vi "Test Calendar.vi"() -> ()   [LabVIEW 2015, in "Calendar.lvclass"]
uses:
  Calendar.lvclass
  DaysOfWeek.ctl
  Read ColorCalendarBackground.vi
  Read ColorCalendarSelectionBackground.vi
  Read ColorCalendarSelectionText.vi
  Read ColorCalendarText.vi
  Read ColorDaysOfWeekBackground.vi
  Read ColorDaysOfWeekText.vi
  Read ColorSelectorBackground.vi
  Read ColorSelectorText.vi
  Read FirstDayOfWeek.vi
  Read VisibleMonthYearSelect.vi
  Read VisibleTodaySelector.vi
  Read VisibleHorizontalLines.vi
  Read VisibleVerticalLines.vi
  Write ColorSelectorBackground.vi
  Write ColorDaysOfWeekText.vi
  Write ColorDaysOfWeekBackground.vi
  Write ColorSelectorText.vi
  Write ColorCalendarText.vi
  Write ColorCalendarBackground.vi
  Write ColorCalendarSelectionBackground.vi
  Write ColorCalendarSelectionText.vi
  Write VisibleTodaySelector.vi
  Write VisibleMonthYearSelect.vi
  Write FirstDayOfWeek.vi
  Write VisibleHorizontalLines.vi
  Write VisibleVerticalLines.vi
panel:
  in  "Veritcal Lines Visible":bool
  in  "Horizontal Lines Visible":bool
  in  "First Day Of Week":T1
  in  "Month-Year Selector Visible":bool
  in  "Today Selector Visible":bool
  in  "Calendar Selection Text":u32(colorbox)
  in  "Calendar Selection Background":u32(colorbox)
  in  "Calendar Background":u32(colorbox)
  in  "Calendar Text":u32(colorbox)
  in  "Selector Text":u32(colorbox)
  in  "Days of Week Background":u32(colorbox)
  in  "Days of Week Text":u32(colorbox)
  in  "Selector Background":u32(colorbox)
  out "Date Output":timestamp format="%<%A, \n%B %d, %Y>T"
  in  "Calendar":T2={"Calendar"=0, "Month"=0, "Year"=1905, "Today Button"=FALSE, "Previous Month"=FALSE, "Next Month"=FALSE, "Cal Overlay"=FALSE, "Year Selection Underlay"=FALSE} {"Year" min=1600 max=3000; "Month" items=["January", "February", "March", "April", "May", "June", "July", "August", "September", "October", "November", "December"]}
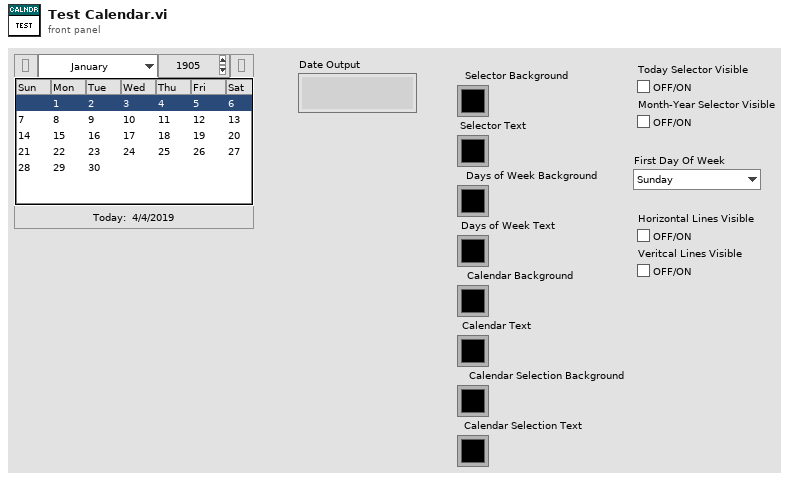
[diagram p1: front panel]
types:
  T1 = typedef "Calendar.lvclass/DaysOfWeek.ctl" = enum16{"Sunday", "Monday", "Tuesday", "Wednesday", "Thursday", "Friday", "Saturday"}
  T2 = cluster{"Calendar":i32, "Month":u16, "Year":i32, "Today Button":bool, "Previous Month":bool, "Next Month":bool, "Cal Overlay":bool, "Year Selection Underlay":bool}
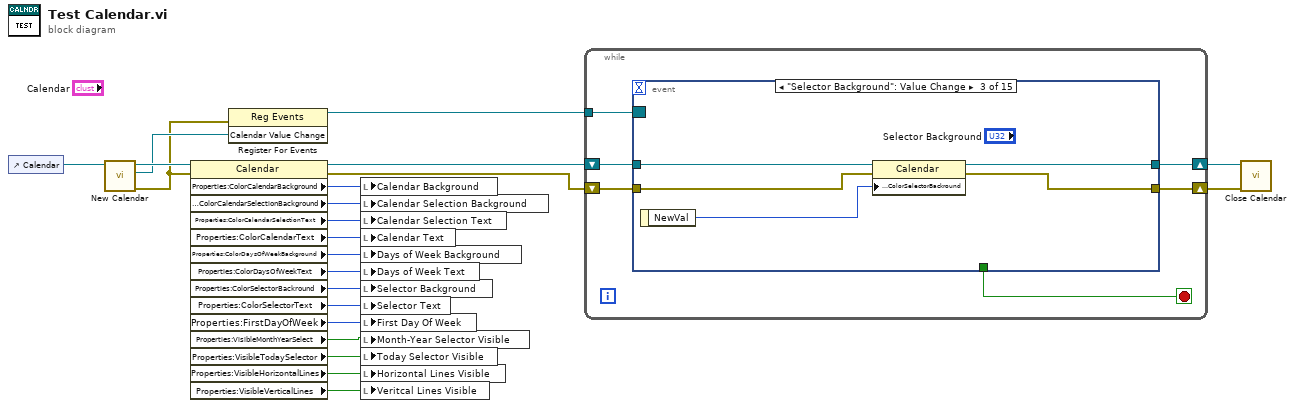
[diagram p0: block diagram]
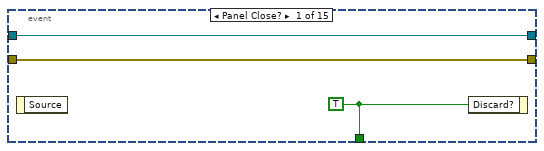
[diagram p2: hidden frame]
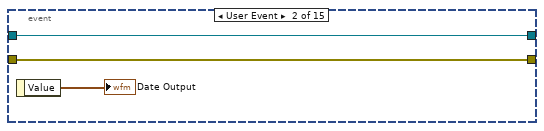
[diagram p3: hidden frame]
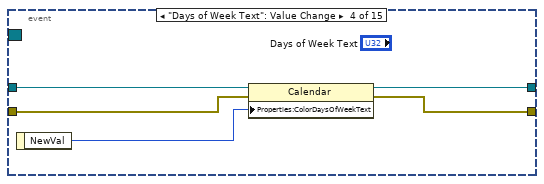
[diagram p4: hidden frame]
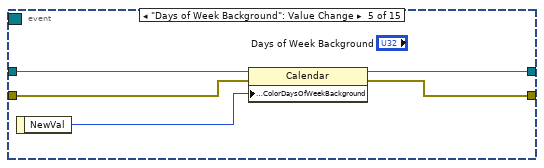
[diagram p5: hidden frame]
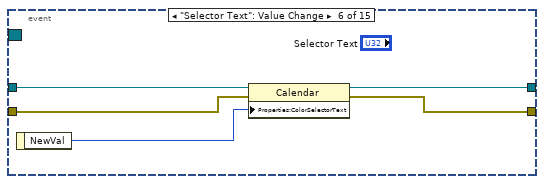
[diagram p6: hidden frame]
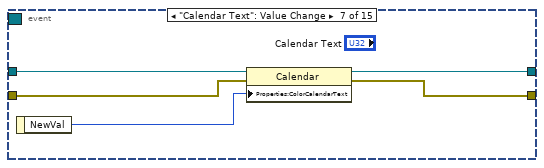
[diagram p7: hidden frame]
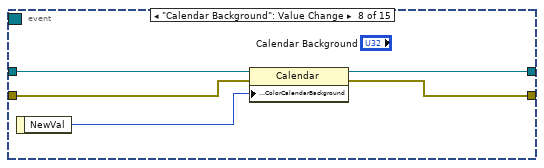
[diagram p8: hidden frame]
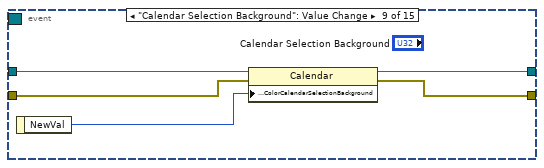
[diagram p9: hidden frame]
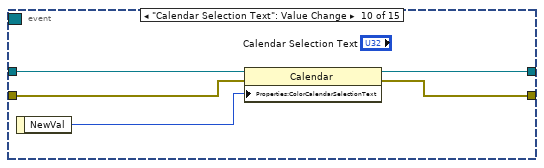
[diagram p10: hidden frame]
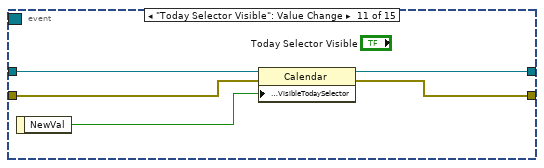
[diagram p11: hidden frame]
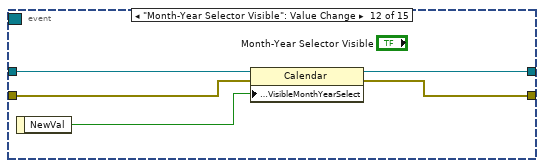
[diagram p12: hidden frame]
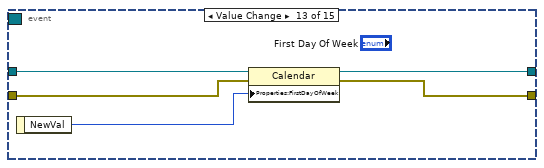
[diagram p13: hidden frame]
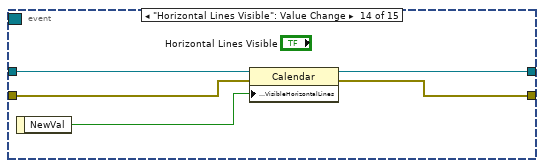
[diagram p14: hidden frame]
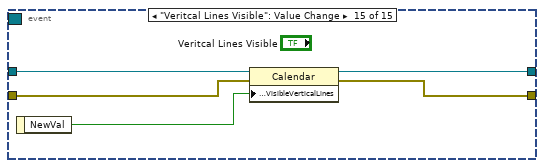
[diagram p15: hidden frame]
diagram:
  n1 = control-ref of="Calendar"() -> (w22:refnum<vi>)
  n2 = call "New Calendar.vi"("Reference"=w22) -> ("error out"=w2:errorcluster, "Calendar Value Change"=w3:refnum<user-event>, "Calendar out"=w18:refnum<class "Calendar.lvclass">)  [unwired: 8 in]
  n3 = property class="Calendar"(reference=w18, error in=w2) -> (reference out=w17:refnum<class "Calendar.lvclass">, error out=w19:errorcluster, "Properties:ColorCalendarBackground"=w16:u32, "Properties:ColorCalendarSelectionBackground"=w15:u32, "Properties:ColorCalendarSelectionText"=w14:u32, "Properties:ColorCalendarText"=w13:u32, "Properties:ColorDaysOfWeekBackground"=w12:u32, "Properties:ColorDaysOfWeekText"=w11:u32, "Properties:ColorSelectorBackround"=w10:u32, "Properties:ColorSelectorText"=w9:u32, "Properties:FirstDayOfWeek"=w8:T1, "Properties:VisibleMonthYearSelect"=w7:bool, "Properties:VisibleTodaySelector"=w6:bool, "Properties:VisibleHorizontalLines"=w5:bool, "Properties:VisibleVerticalLines"=w4:bool)
  n4 = register-events(error in=w2, w3) -> (reference out=w1:refnum<event-registration>)  [unwired: 1 in, 1 out]
  n5 = local write "Calendar Background"(w16) -> ()
  n6 = local write "Calendar Selection Background"(w15) -> ()
  n7 = local write "Calendar Selection Text"(w14) -> ()
  n8 = local write "Calendar Text"(w13) -> ()
  n9 = local write "Days of Week Background"(w12) -> ()
  n10 = local write "Days of Week Text"(w11) -> ()
  n11 = local write "Selector Background"(w10) -> ()
  n12 = local write "Selector Text"(w9) -> ()
  n13 = local write "First Day Of Week"(w8) -> ()
  n14 = local write "Month-Year Selector Visible"(w7) -> ()
  n15 = local write "Today Selector Visible"(w6) -> ()
  n16 = local write "Horizontal Lines Visible"(w5) -> ()
  n17 = local write "Veritcal Lines Visible"(w4) -> ()
  n18 = while {
    shift-right: [w27] -> w21
    shift-left: w17 -> [w26]
    shift-right: [w24] -> w20
    shift-left: w19 -> [w25]
    tunnel: w1 -> [w23]
    stop <- w28 stop-if-true
    n19 = event shown="[2] \"Selector Background\": Value Change" {
      selector: w23 -> [_ _ _ _ _ _ _ _ _ _ _ _ _ _ _]
      dyn-events: _ -> [_ _ _ _ _ _ _ _ _ _ _ _ _ _ _]
      timeout: _ -> [_ _ _ _ _ _ _ _ _ _ _ _ _ _ _]
      tunnel: [w31 _ _ _ _ _ _ _ _ _ _ _ _ _ _] -> w28
      tunnel: [w30 w34 w36 w41 w46 w51 w56 w61 w66 w71 w76 w81 w86 w91 w96] -> w27
      tunnel: w26 -> [w30 w34 w39 w44 w49 w54 w59 w64 w69 w74 w79 w84 w89 w94 w99]
      tunnel: w25 -> [w29 w32 w38 w43 w48 w53 w58 w63 w68 w73 w78 w83 w88 w93 w98]
      tunnel: [w29 w32 w35 w40 w45 w50 w55 w60 w65 w70 w75 w80 w85 w90 w95] -> w24
      event Panel Close? {
        w31 = TRUE
        n20 = event-data() -> ()  [unwired: 1 in, 1 out]
        n21 = event-data("Discard?"=w31) -> ()  [unwired: 1 in, 1 out]
      }
      event User Event {
        n22 = event-data() -> ("Value"=→"Date Output":timestamp)  [unwired: 1 in]
      }
      event "Selector Background": Value Change {
        n23 = event-data() -> ("NewVal"=w37:u32)  [unwired: 1 in]
        n24 = property class="Calendar"(reference=w39, error in=w38, "Properties:ColorSelectorBackround"=w37) -> (reference out=w36:refnum<class "Calendar.lvclass">, error out=w35:errorcluster)
      }
      event "Days of Week Text": Value Change {
        n25 = event-data() -> ("NewVal"=w42:u32)  [unwired: 1 in]
        n26 = property class="Calendar"(reference=w44, error in=w43, "Properties:ColorDaysOfWeekText"=w42) -> (reference out=w41:refnum<class "Calendar.lvclass">, error out=w40:errorcluster)
      }
      event "Days of Week Background": Value Change {
        n27 = event-data() -> ("NewVal"=w47:u32)  [unwired: 1 in]
        n28 = property class="Calendar"(reference=w49, error in=w48, "Properties:ColorDaysOfWeekBackground"=w47) -> (reference out=w46:refnum<class "Calendar.lvclass">, error out=w45:errorcluster)
      }
      event "Selector Text": Value Change {
        n29 = event-data() -> ("NewVal"=w52:u32)  [unwired: 1 in]
        n30 = property class="Calendar"(reference=w54, error in=w53, "Properties:ColorSelectorText"=w52) -> (reference out=w51:refnum<class "Calendar.lvclass">, error out=w50:errorcluster)
      }
      event "Calendar Text": Value Change {
        n31 = event-data() -> ("NewVal"=w57:u32)  [unwired: 1 in]
        n32 = property class="Calendar"(reference=w59, error in=w58, "Properties:ColorCalendarText"=w57) -> (reference out=w56:refnum<class "Calendar.lvclass">, error out=w55:errorcluster)
      }
      event "Calendar Background": Value Change {
        n33 = event-data() -> ("NewVal"=w62:u32)  [unwired: 1 in]
        n34 = property class="Calendar"(reference=w64, error in=w63, "Properties:ColorCalendarBackground"=w62) -> (reference out=w61:refnum<class "Calendar.lvclass">, error out=w60:errorcluster)
      }
      event "Calendar Selection Background": Value Change {
        n35 = event-data() -> ("NewVal"=w67:u32)  [unwired: 1 in]
        n36 = property class="Calendar"(reference=w69, error in=w68, "Properties:ColorCalendarSelectionBackground"=w67) -> (reference out=w66:refnum<class "Calendar.lvclass">, error out=w65:errorcluster)
      }
      event "Calendar Selection Text": Value Change {
        n37 = event-data() -> ("NewVal"=w72:u32)  [unwired: 1 in]
        n38 = property class="Calendar"(reference=w74, error in=w73, "Properties:ColorCalendarSelectionText"=w72) -> (reference out=w71:refnum<class "Calendar.lvclass">, error out=w70:errorcluster)
      }
      event "Today Selector Visible": Value Change {
        n39 = event-data() -> ("NewVal"=w77:bool)  [unwired: 1 in]
        n40 = property class="Calendar"(reference=w79, error in=w78, "Properties:VisibleTodaySelector"=w77) -> (reference out=w76:refnum<class "Calendar.lvclass">, error out=w75:errorcluster)
      }
      event "Month-Year Selector Visible": Value Change {
        n41 = event-data() -> ("NewVal"=w82:bool)  [unwired: 1 in]
        n42 = property class="Calendar"(reference=w84, error in=w83, "Properties:VisibleMonthYearSelect"=w82) -> (reference out=w81:refnum<class "Calendar.lvclass">, error out=w80:errorcluster)
      }
      event Value Change {
        n43 = event-data() -> ("NewVal"=w87:T1)  [unwired: 1 in]
        n44 = property class="Calendar"(reference=w89, error in=w88, "Properties:FirstDayOfWeek"=w87) -> (reference out=w86:refnum<class "Calendar.lvclass">, error out=w85:errorcluster)
      }
      event "Horizontal Lines Visible": Value Change {
        n45 = event-data() -> ("NewVal"=w92:bool)  [unwired: 1 in]
        n46 = property class="Calendar"(reference=w94, error in=w93, "Properties:VisibleHorizontalLines"=w92) -> (reference out=w91:refnum<class "Calendar.lvclass">, error out=w90:errorcluster)
      }
      event "Veritcal Lines Visible": Value Change {
        n47 = event-data() -> ("NewVal"=w97:bool)  [unwired: 1 in]
        n48 = property class="Calendar"(reference=w99, error in=w98, "Properties:VisibleVerticalLines"=w97) -> (reference out=w96:refnum<class "Calendar.lvclass">, error out=w95:errorcluster)
      }
    }
  }
  n49 = call "Close Calendar.vi"("error in (no error)"=w20, "Calendar in"=w21) -> ()  [unwired: 9 in, 1 out]
